vi "Delete Linked List.vi"(8 "error in (no error)":errorcluster, 10 "Linked List ID":string, 11 "Linked List Ref":refnum<data-value>) -> (0 "error out":errorcluster, 3 "Linked List Ref out":refnum<data-value>)   [LabVIEW 2020, in "Linked Lists.lvlib" / "Linked List Ref.lvclass"]
uses:
  <vilib>/gpm_packages/@cs/linked-list/Source/Linked List/Linked List Ref/Linked List Ref.lvclass
  <vilib>/gpm_packages/@cs/linked-list/Source/Linked List/ILinkedList/ILinked List.lvclass
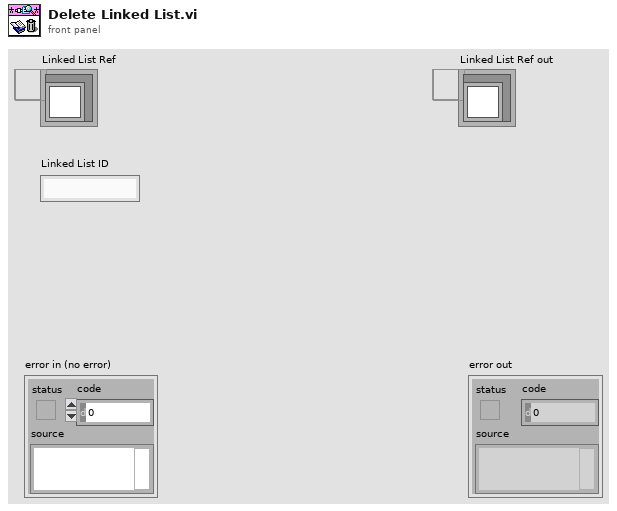
[diagram p1: front panel]
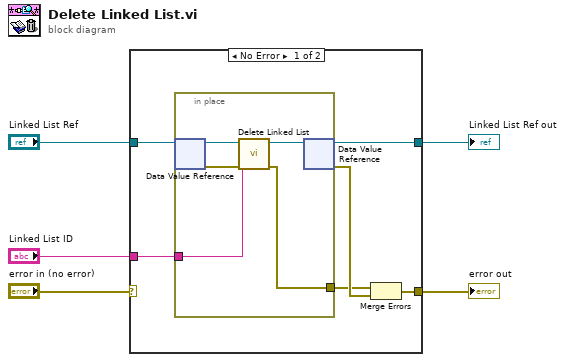
[diagram p0: block diagram]
diagram:
  n1 = case shown="No Error" "error in (no error)" {
    selector: "error in (no error)" -> [_ w18]
    tunnel: "Linked List Ref" -> [w11 w17]
    tunnel: "Linked List ID" -> [w10 _]
    tunnel: [w9 w17] -> w3
    tunnel: [w7 w18] -> w1
    frame No Error {
      n2 = in-place {
        in-place-border: w10 -> [w14]
        in-place-border: [w12] -> w6
        n3 = in-place-dvr #1(w11) -> (w16:refnum<class "ILinked List.lvclass">, w15:errorcluster)
        n4 = call-dynamic "Delete Linked List.vi"("error in (no error)"=w15, "Unique ID"=w14, "ILinked List in"=w16) -> ("error out"=w12:errorcluster, "ILinked List out"=w13:refnum<class "ILinked List.lvclass">)  [unwired: 7 in]
        n5 = in-place-dvr #1(w13) -> (w9:refnum<data-value>, w8:errorcluster)
      }
      n6 = Merge Errors(w6, w8) -> (w7:errorcluster)
    }
    frame Error {
    }
  }
  "error out" <- w1
  "Linked List Ref out" <- w3
